vi "Initialize.vi"(6 "Actor Name":string, 7 "Host Name":string, 8 "error in (no error)":errorcluster, 10 "Application Data":path, 11 "Message Broker":refnum<class "Message Broker Interface Ref.lvclass">) -> (0 "error out":errorcluster, 3 "Terminal Menus out":refnum<class "Terminal Menus.lvclass">)   [LabVIEW 2016, in "CLD Exam - ATM.lvlib" / "Terminal Menus.lvclass"]
uses:
  Terminal Menus.lvclass
  Mediator/Classes/Message Broker Interface Ref/Message Broker Interface Ref.lvclass
  D:/Repos/Stream/software/Mediator/Classes/Message Broker Interface/Message Broker Interface.lvclass
  Terminal Menus.lvclass/Terminal Menus.ctl
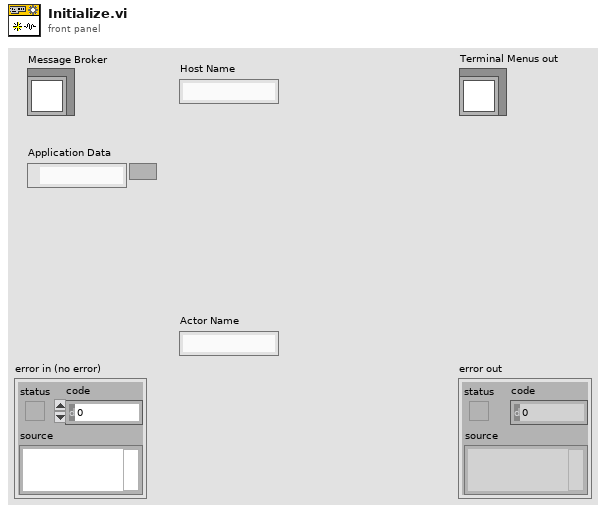
[diagram p1: front panel]
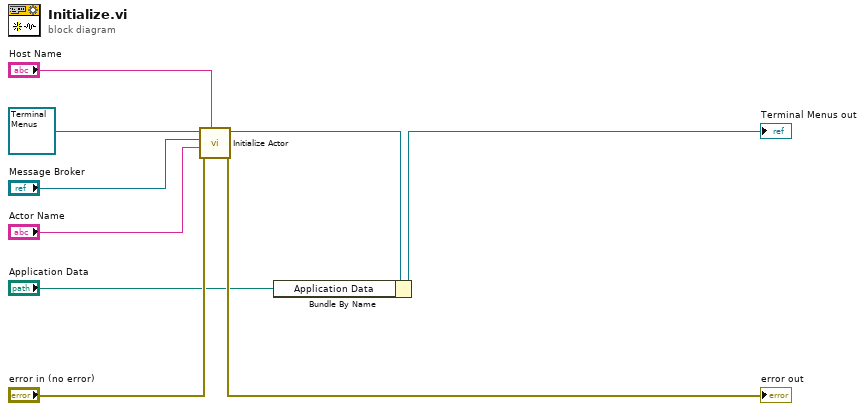
[diagram p0: block diagram]
diagram:
  n1 = call-dynamic "Initialize Actor.vi"("Host Name"="Host Name", "error in (no error)"="error in (no error)", "Actor Name"="Actor Name", "Message Broker Interface"="Message Broker", "Terminal Menus in"=refnum<class "Terminal Menus.lvclass"> refnum) -> ("error out"=→"error out":errorcluster, "Terminal Menus out"=w3:refnum<class "Terminal Menus.lvclass">)  [unwired: 5 in]
  n2 = Bundle By Name(cluster=w3, "Application Data"="Application Data") -> (→"Terminal Menus out":refnum<class "Terminal Menus.lvclass">)
